vi "SIM Adams Eval Error Core.vi"(0 "outputs":dbl[](array[numeric]), 1 "min float":dbl, 2 "Delta Method Order":i32, 3 "max step ratio":dbl, 5 "step size":dbl, 7 "proposed step size":dbl, 9 "min step size":dbl, 11 "Adams data":T1, 12 "max step size":dbl, 13 "relative tolerance":dbl, 14 "absolute tolerance":dbl) -> (4 "outputs out":dbl[](array[numeric]), 6 "step accepted? out":bool, 8 "proposed step size out":dbl, 10 "proposed max step ratio":dbl, 15 "Adams data out":T1)   [LabVIEW 2024]
uses:
  SIM Adams data.ctl
  SIM Adams stages.ctl
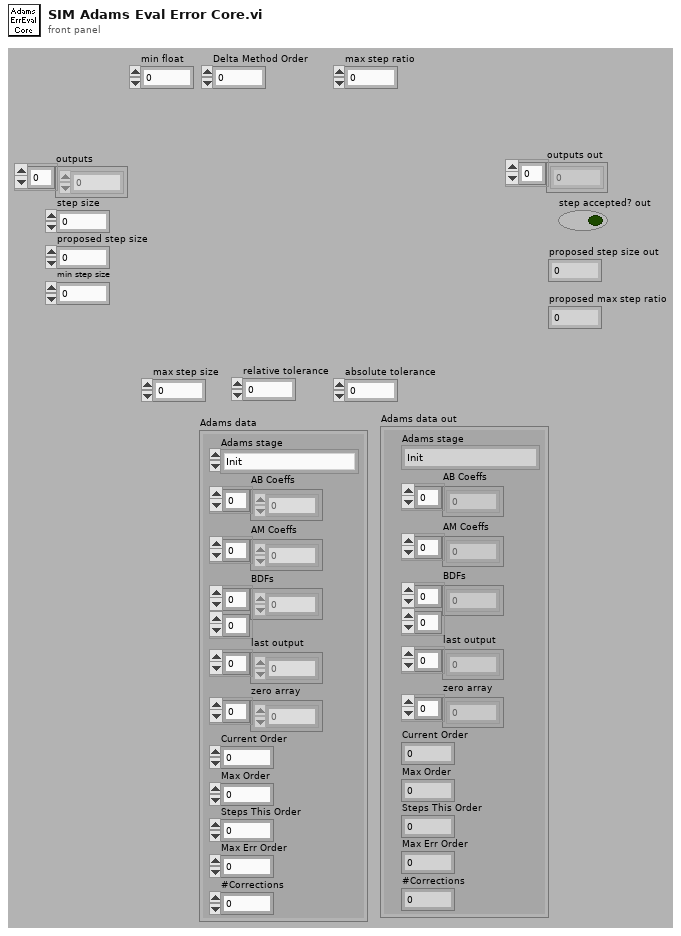
[diagram p1: front panel]
types:
  T1 = typedef "SIM Adams data.ctl" = cluster{"Adams stage":T2, "AB Coeffs":dbl[], "AM Coeffs":dbl[], "BDFs":dbl[][], "last output":dbl[], "zero array":dbl[], "Current Order":i32, "Max Order":i32, "Steps This Order":i32, "Max Err Order":i32, "#Corrections":i32}
  T2 = typedef "SIM Adams stages.ctl" = enum16{"Init", "Predict", "Correct", "Eval Error", "Choose StepSize", "Reset BDFs"}
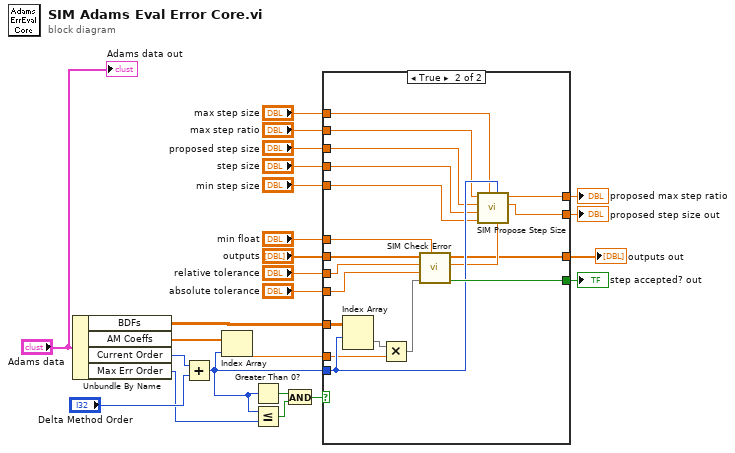
[diagram p0: block diagram]
diagram:
  n1 = Unbundle By Name("Adams data") -> ("BDFs"=w18:dbl[][], "AM Coeffs"=w13:dbl[], "Current Order"=w15:i32, "Max Err Order"=w14:i32)
  n2 = Add(x=w15, y="Delta Method Order") -> (x+y=w1:i32)
  n3 = Index Array(array=w13, index=w1) -> (element=w2:dbl)
  n4 = Greater Than 0?(x=w1) -> (x > 0?=w21:bool)
  n5 = Less Or Equal?(x=w1, y=w14) -> (x <= y?=w17:bool)
  n6 = And(x=w21, y=w17) -> (x .and. y?=w20:bool)
  n7 = case shown="True" w20 {
    tunnel: "outputs" -> [w25 w29]
    tunnel: w18 -> [_ w44]
    tunnel: w1 -> [_ w37]
    tunnel: [_ w38] -> w24
    tunnel: [_ w35] -> w23
    tunnel: [_ w36] -> w22
    tunnel: "relative tolerance" -> [_ w41]
    tunnel: "min float" -> [_ w42]
    tunnel: "absolute tolerance" -> [_ w40]
    tunnel: "max step size" -> [_ w34]
    tunnel: "max step ratio" -> [_ w33]
    tunnel: "proposed step size" -> [_ w32]
    tunnel: "step size" -> [_ w31]
    tunnel: "min step size" -> [_ w30]
    tunnel: [w25 w27] -> w3
    tunnel: w2 -> [_ w26]
    frame False {
    }
    frame True {
      n8 = Index Array(array=w44, index (row)=w37) -> (element=w43:dbl[])  [unwired: 1 in]
      n9 = Multiply(x=w43, y=w26) -> (x*y=w39:dbl[])
      n10 = call "SIM Check Error.vi"("min float"=w42, "estimated error"=w39, "absolute tolerance"=w40, "relative tolerance"=w41, "Solution"=w29) -> ("within acceptable err?"=w38:bool, "acceptable err/estimated err"=w28:dbl, "Solution Out"=w27:dbl[])  [unwired: 4 out]
      n11 = call "SIM Propose Step Size.vi"("acceptable err/estimated err"=w28, "error order"=w37, "max step size"=w34, "min step size"=w30, "step size"=w31, "proposed step size"=w32, "max step ratio"=w33) -> ("proposed step size out"=w35:dbl, "proposed max step ratio"=w36:dbl)  [unwired: 3 out]
    }
  }
  "step accepted? out" <- w24
  "proposed step size out" <- w23
  "proposed max step ratio" <- w22
  "outputs out" <- w3
  "Adams data out" <- "Adams data"
